vi "AdaptToInputs.vi"(3 "Term Types":T1, 4 "XRef":refnum<vi>, 5 "State In":T5) -> (0 "Reply":string[](array[string]), 2 "State Out":T5)   [LabVIEW 2012, in "ConPane Wrapper.xnode"]
uses:
  ConPane Wrapper.xnode
  State.ctl
  <vilib>/picture/picture.llb/imagedata.ctl
  <vilib>/XNodeSupport/XNodeTerm3Array.ctl
  <vilib>/XNodeSupport/XNodeTerm3.ctl
  <vilib>/XNodeSupport/XNodeString.ctl
  <vilib>/XNodeSupport/XNodeVariant.ctl
  <vilib>/XNodeSupport/XNodeRect32.ctl
  <vilib>/XNodeSupport/XNodeInt.ctl
  <vilib>/XNodeSupport/XNodeBool.ctl
  <vilib>/XNodeSupport/XNodeTermDirection.ctl
  Subvis/Term Types.ctl
  Subvis/Term Type.ctl
  <vilib>/XNodeSupport/XNodeTermTypeIDPairs.ctl
  <vilib>/XNodeSupport/XNodeTermTypeIDPair.ctl
  <vilib>/XNodeSupport/XNodeType.ctl
  <vilib>/XNodeSupport/NI_XNodeSupport.lvlib
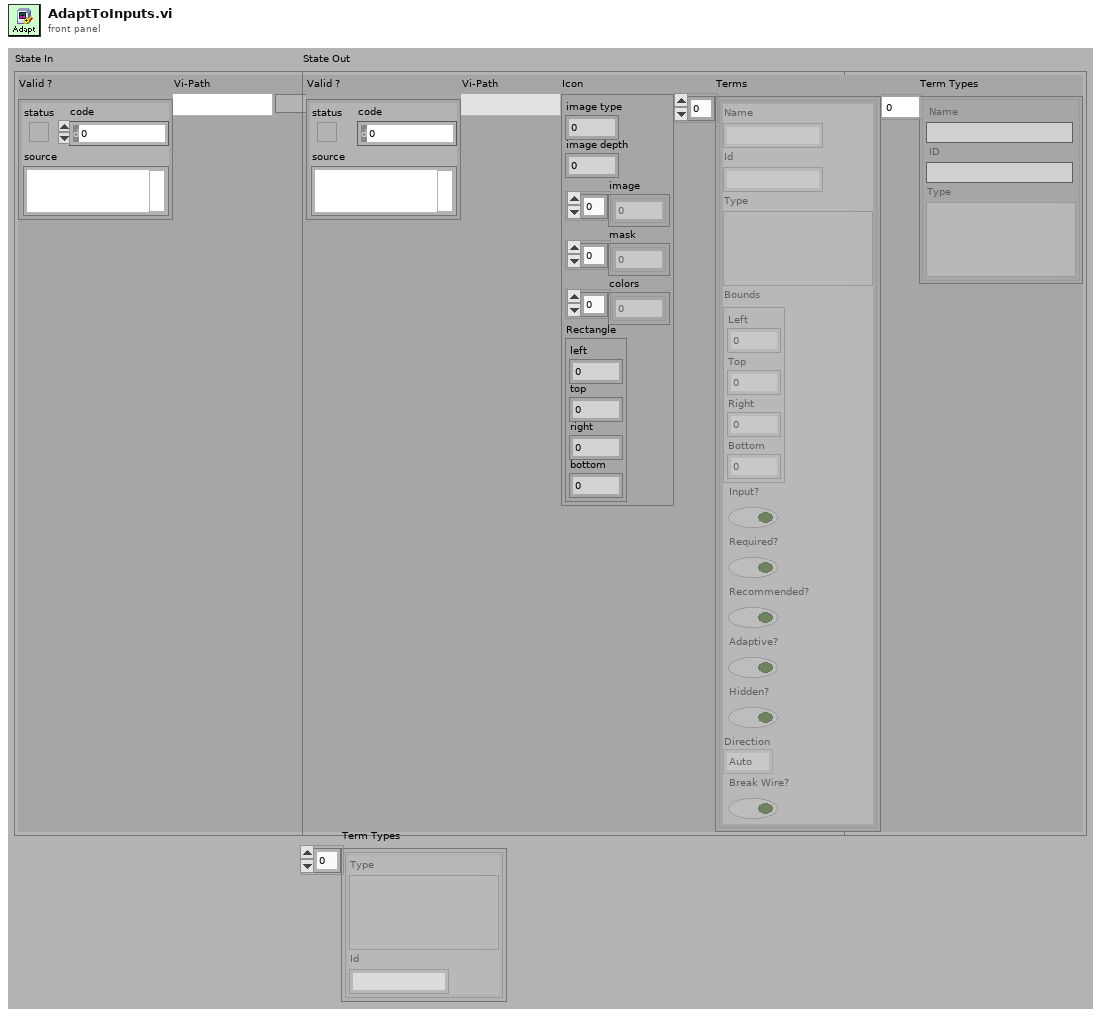
[diagram p1: front panel]
types:
  T1 = typedef "NI_XNodeSupport.lvlib/XNodeTermTypeIDPairs.ctl" = T2[]
  T2 = typedef "NI_XNodeSupport.lvlib/XNodeTermTypeIDPair.ctl" = cluster{"Type":T3, "Id":T4}
  T3 = typedef "NI_XNodeSupport.lvlib/XNodeType.ctl" = variant
  T4 = typedef "NI_XNodeSupport.lvlib/XNodeString.ctl" = string
  T5 = typedef "ConPane Wrapper.xnode/State.ctl" = cluster{"Valid ?":errorcluster, "Vi-Path":path, "Icon":T6, "Terms":T7, "Term Types":T14}
  T6 = typedef "imagedata.ctl" = cluster{"image type":i32, "image depth":i32, "image":u8[], "mask":u8[], "colors":u32[], "Rectangle":cluster{"left":i16, "top":i16, "right":i16, "bottom":i16}}
  T7 = typedef "NI_XNodeSupport.lvlib/XNodeTerm3Array.ctl" = T8[]
  T8 = typedef "NI_XNodeSupport.lvlib/XNodeTerm3.ctl" = cluster{"Name":T4, "Id":T4, "Type":T9, "Bounds":T10, "Input?":T12, "Required?":T12, "Recommended?":T12, "Adaptive?":T12, "Hidden?":T12, "Direction":T13, "Break Wire?":T12}
  T9 = typedef "NI_XNodeSupport.lvlib/XNodeVariant.ctl" = variant
  T10 = typedef "NI_XNodeSupport.lvlib/XNodeRect32.ctl" = cluster{"Left":T11, "Top":T11, "Right":T11, "Bottom":T11}
  T11 = typedef "NI_XNodeSupport.lvlib/XNodeInt.ctl" = i32
  T12 = typedef "NI_XNodeSupport.lvlib/XNodeBool.ctl" = bool
  T13 = typedef "NI_XNodeSupport.lvlib/XNodeTermDirection.ctl" = enum32{"Auto", "Up", "Down", "Left", "Right", "Center"}
  T14 = typedef "Term Types.ctl" = T15[]
  T15 = typedef "Term Type.ctl" = cluster{"Name":string, "ID":string, "Type":variant}
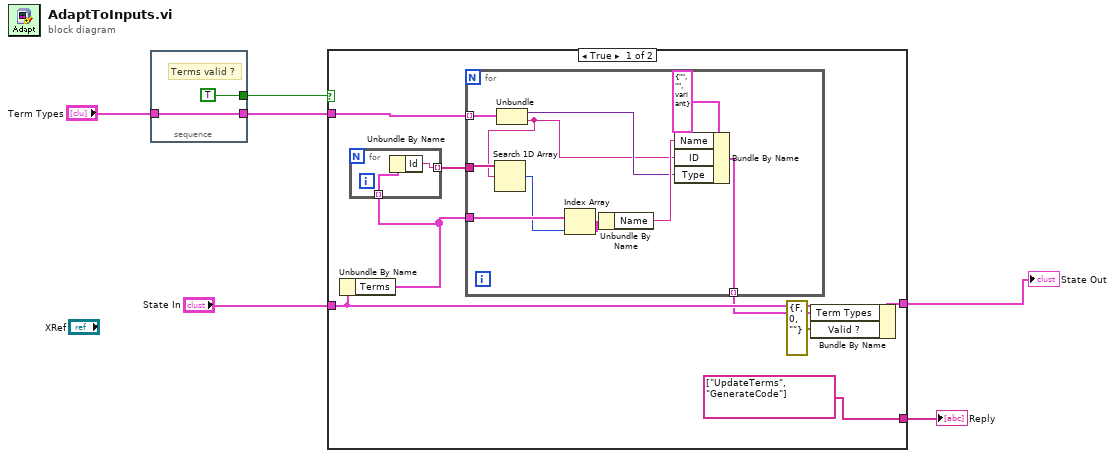
[diagram p0: block diagram]
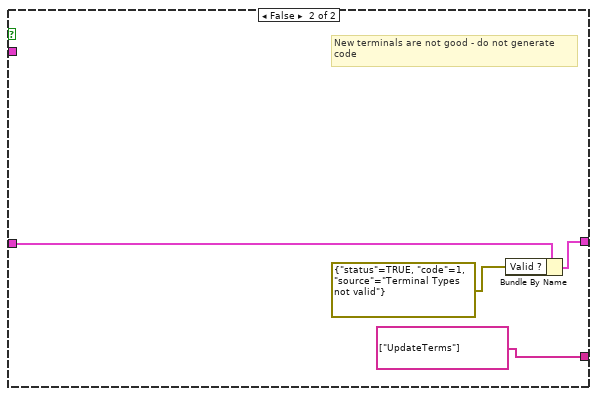
[diagram p2: hidden frame]
diagram:
  n1 = stacked-sequence {
    tunnel: "Term Types" -> [w8]
    tunnel: [w8] -> w4
    tunnel: [TRUE] -> w5
    frame #0 {
      # "Terms valid ?"
    }
  }
  n2 = case shown="True" w5 {
    tunnel: w4 -> [w12 _]
    tunnel: "State In" -> [w13 w32]
    tunnel: [w15 w30] -> w2
    tunnel: [string[] ["UpdateTerms", "GenerateCode"] ("Reply") string[] ["UpdateTerms"] ("Reply")] -> w1
    frame True {
      n3 = Unbundle By Name(w13) -> ("Terms"=w10:T7)
      n4 = for {
        tunnel: w10 -> [w18] mode=indexing
        tunnel: [w17] -> w9 mode=indexing
        n5 = Unbundle By Name(w18) -> ("Id"=w17:T4)
      }
      n6 = for {
        tunnel: w12 -> [w28] mode=indexing
        tunnel: w10 -> [w27]
        tunnel: [w22] -> w11 mode=indexing
        tunnel: w9 -> [w21]
        n7 = Unbundle(w28) -> ("Type"=w23:T3, "Id"=w20:T4)
        n8 = Search 1D Array(1D array=w21, element=w20) -> (index of element=w19:i32)  [unwired: 1 out]
        n9 = Index Array(array=w27, index=w19) -> (element=w26:T8)
        n10 = Unbundle By Name(w26) -> ("Name"=w24:T4)
        n11 = Bundle By Name(cluster=T15 {"Name"="", "ID"="", "Type"=variant} ("Term Type"), "Name"=w24, "ID"=w20, "Type"=w23) -> (w22:T15)
      }
      n12 = Bundle By Name(cluster=w13, "Term Types"=w11, "Valid ?"=errorcluster {"status"=FALSE, "code"=0, "source"=""}) -> (w15:T5)
    }
    frame False {
      # "New terminals are not good - do not generate\ncode"
      n13 = Bundle By Name(cluster=w32, "Valid ?"=errorcluster {"status"=TRUE, "code"=1, "source"="Terminal Types not valid"}) -> (w30:T5)
    }
  }
  "Reply" <- w1
  "State Out" <- w2
